vi "pulse amplitude fitter.vi"() -> ()   [LabVIEW 2016]
uses:
  <vilib>/Analysis/4window.llb/Hanning Window (DBL).vi
  <vilib>/Analysis/baseanly.llb/Real Dot Product.vi
  <vilib>/Analysis/baseanly.llb/Mean (DBL).vi
  <vilib>/Analysis/4window.llb/AllCosWindow (DBL).vi
  subs/path list.vi
  subs/global mass.vi
  <vilib>/Analysis/NI_AALPro.lvlib
  <vilib>/Analysis/NI_AALBase.lvlib
panel:
  in  "experiment":u16(ring) items=["2D SdH", "2D dHvA (dM/dt)", "2D dHvA (dM/dB)", "2D dHvA (M)", "2D dHvA (torque)", "3D SdH", "3D dHvA (dM/dt)", "3D dHvA (dM/dB)", "3D dHvA (M)", "3D dHvA (torque)"]
  in  "save parameters?":bool
  in  "save plots?":bool
  in  "format":string="%.6e"
  in  "?":bool
  in  "renomalise\namplitudes?":dbl[](array[numeric]) format="%.2f"
  out "fitted intercept":dbl[][](array[numeric]) format="%.2f"
  out "fitted m* over all (1/b)":dbl[](array[numeric]) format="%.2f"
  out "fitted gamma":dbl[][](array[numeric]) format="%.2f"
  in  "mass constant":dbl=1.0 format="%.2f"
  in  "Dingle plot mass option":u16(ring) items=["single fitted value", "field dependent", "use mass constant"]
  out "fitted m*":dbl[][](array[numeric]) format="%.2f"
  out "plot parameters":string="1/B   F   m*"
  in  "selection":u16(ring) items=["amp. vs. temperature T", "amp. vs. 1/B"]
  in  "no. points in 1/B":u16(ring) items=["1", "3", "7", "15", "31", "63", "127"]
  in  "frequencies":dbl[](array[numeric]) format="%.2f"
  in  "temperatures":dbl[](array[numeric]) format="%.2f"
  out "plotted data":cluster{"temperatures":dbl[], dbl[]}[](graph)
  in  "type of interpolation":u16(ring) items=["linear", "cubic spline", "polynomial"]
  in  "no. 1/B interpolation points":u16(ring) items=["1024", "2048", "4096", "8192", "16384", "32768"]
  in  "y domain":u16(ring) items=["channel A"]
  in  "x domain":u16(ring) items=["1/B (rising field)", "1/B (falling field)", "1/B (rising field + falling field)", "1/B (rising field - falling field)"]
  # "#\n0\n1\n2\n3\n4\n5\n6\n7\n8\n9\n10\n11\n12\n13\n14\n15\n16\n17\n18\n19\n20\n21\n22\n23\n24\n25\n26\n27\n28\n29\n30"
  # "1/B"
  # "T"
  # "F"
  # "F"
  # "T"
  # "F"
  # "F"
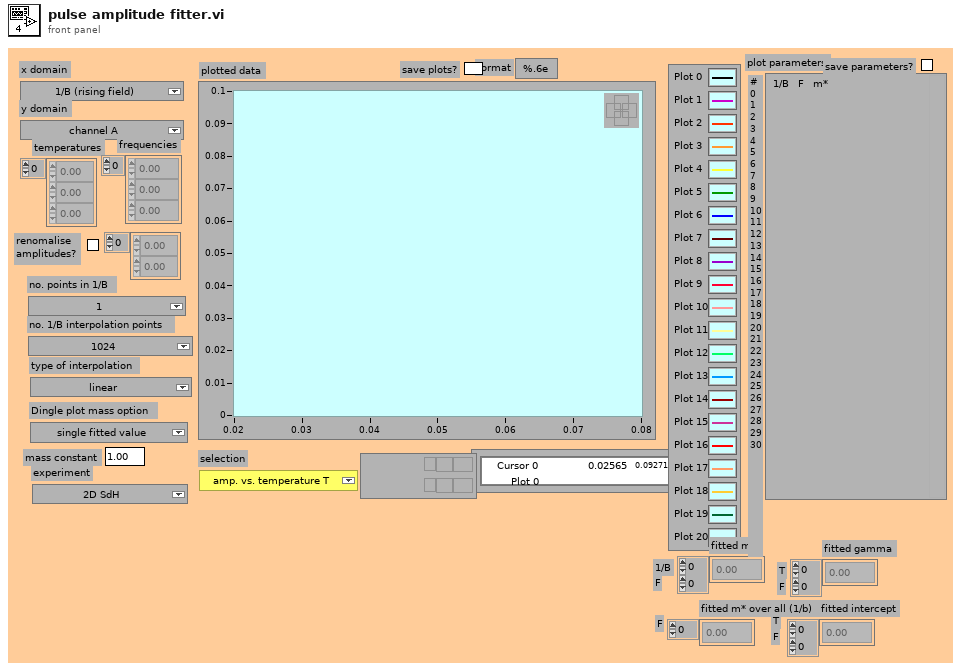
[diagram p1: front panel]
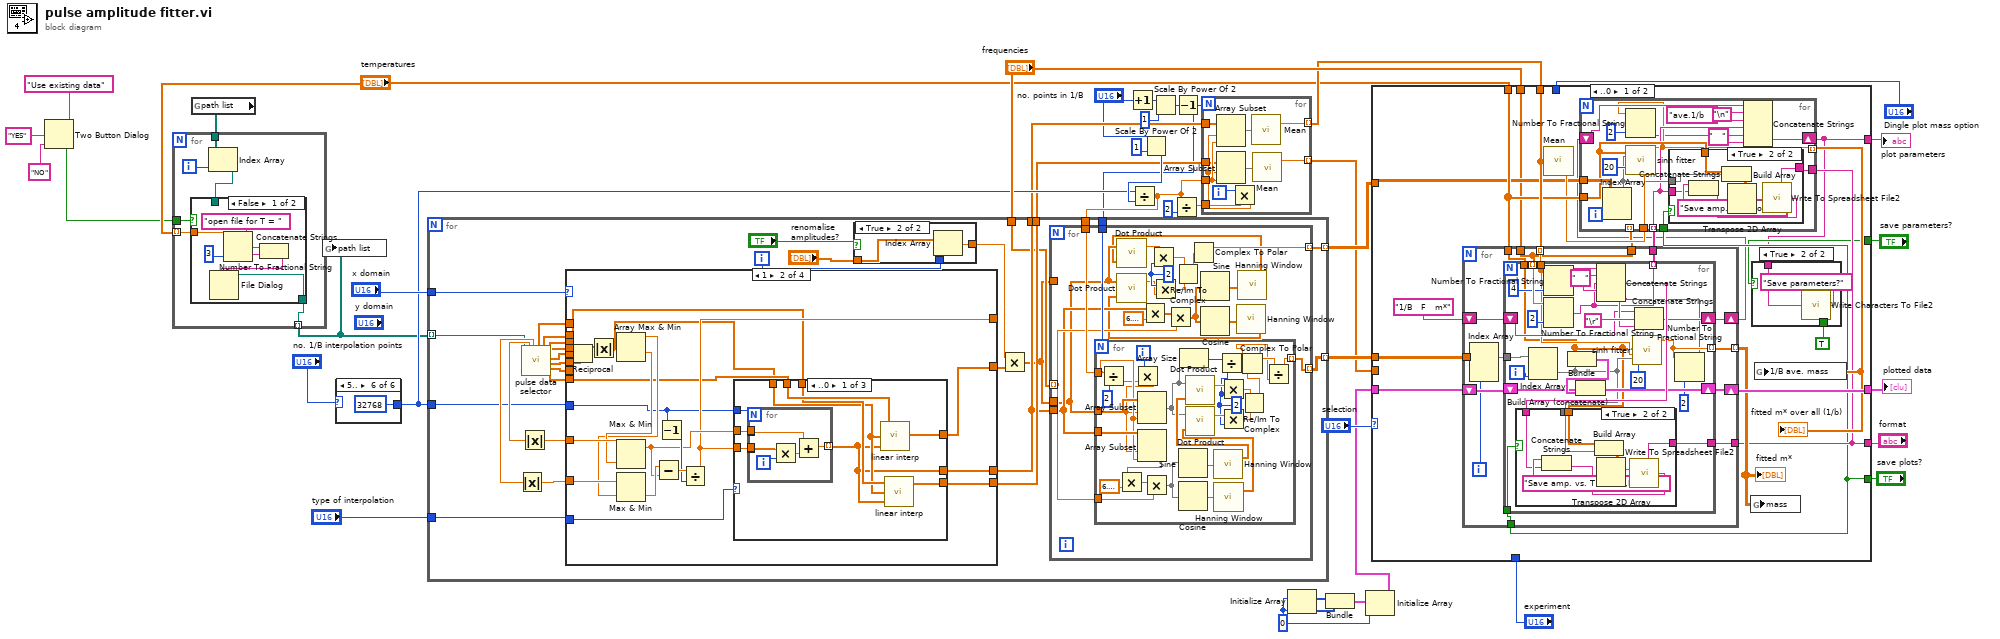
[diagram p0: block diagram]
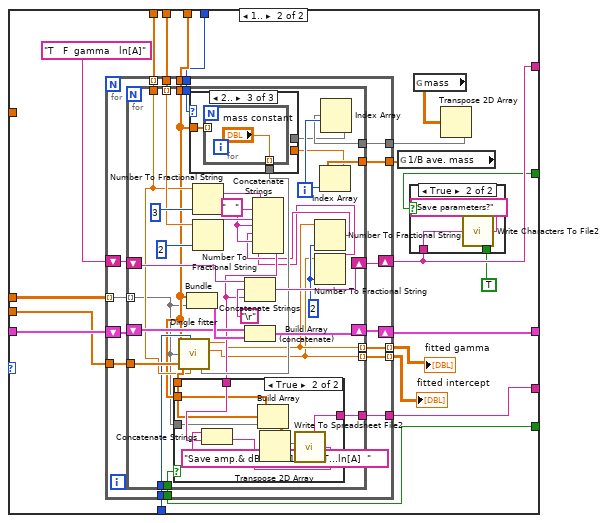
[diagram p6: hidden frame]
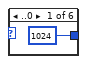
[diagram p11: hidden frame]
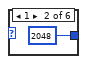
[diagram p12: hidden frame]
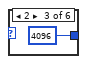
[diagram p13: hidden frame]
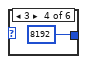
[diagram p14: hidden frame]
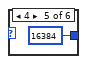
[diagram p15: hidden frame]
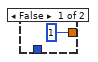
[diagram p16: hidden frame]
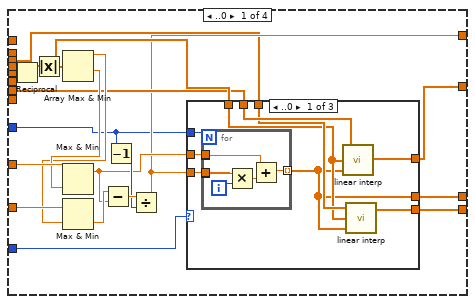
[diagram p17: hidden frame]
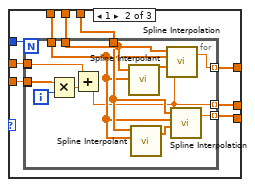
[diagram p18: hidden frame]
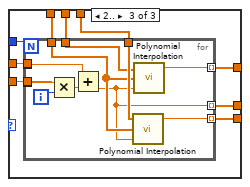
[diagram p19: hidden frame]
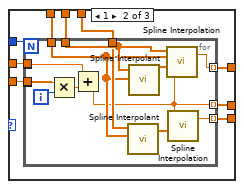
[diagram p20: hidden frame]
diagram:
  w23 = 0
  n1 = Two Button Dialog(message="Use existing data", 1:"NO", 2:"YES") -> (T button?=w8:bool)
  n2 = global read "path list.vi" "path list"() -> (w12:path[])
  n3 = for {
    tunnel: "temperatures" -> [w46] mode=indexing
    tunnel: [w45] -> w13 mode=indexing
    tunnel: w12 -> [w43]
    tunnel: w8 -> [w44]
    i -> [w42]
    n4 = Index Array(array=w43, index=w42) -> (element=w41:path)
    n5 = case shown="False" w44 {
      tunnel: w46 -> [w48 _]
      tunnel: [w47 w53] -> w45
      tunnel: w41 -> [_ w53]
      frame False {
        n6 = Number To Fractional String(number=w48, precision (6)=3) -> (F-format string=w51:string)  [unwired: 2 in]
        n7 = Concatenate Strings("open file for T = ", w51) -> (w52:string)
        n8 = File Dialog(7:w52) -> (3:w47:path)  [unwired: 6 in, 3 out]
      }
      frame True {
      }
    }
  }
  n9 = global write "path list.vi" "path list"(w13) -> ()
  n10 = case shown="5.." "no. 1/B interpolation points" {
    tunnel: [1024 2048 4096 8192 16384 32768] -> w32
    frame ..0 {
    }
    frame 1 {
    }
    frame 2 {
    }
    frame 3 {
    }
    frame 4 {
    }
    frame 5.. {
    }
  }
  n11 = Increment(x="no. points in 1/B") -> (x+1=w36:u16)
  n12 = Scale By Power Of 2(n="no. points in 1/B", x=1) -> (x*2^n=w34:i32)
  n13 = Divide(x=w32, y=w34) -> (x/y=w31:dbl)
  n14 = Scale By Power Of 2(n=w36, x=1) -> (x*2^n=w35:i32)
  n15 = Divide(x=w31, y=2) -> (x/y=w29:dbl)
  n16 = Decrement(x=w35) -> (x-1=w16:i32)
  n17 = for {
    tunnel: "x domain" -> [w70]
    tunnel: w32 -> [w78]
    tunnel: "type of interpolation" -> [w77]
    tunnel: [w76] -> w25 mode=indexing
    tunnel: "frequencies" -> [w67]
    tunnel: w31 -> [w73]
    tunnel: [w68] -> w28
    tunnel: [w72] -> w27
    tunnel: w16 -> [w71]
    tunnel: w13 -> [w69] mode=indexing
    tunnel: [w66] -> w7 mode=indexing
    i -> [w63]
    n18 = call "pulse data selector.vi"("file path (dialog if empty)"=w69) -> ("1/B start interpolation"=w83:dbl, "1/B end interpolation"=w84:dbl, "time rising"=w79:dbl[], "time falling"=w80:dbl[], "dB/dt rising"=w75:dbl[], "dB/dt falling"=w74:dbl[], "B rising"=w87:dbl[], "B falling"=w88:dbl[], "ch A rising"=w81:dbl[], "ch A falling"=w82:dbl[])  [unwired: 6 in, 3 out]
    n19 = Absolute Value(x=w84) -> (abs(x)=w86:dbl)
    n20 = Absolute Value(x=w83) -> (abs(x)=w85:dbl)
    n21 = case shown="1" w70 {
      tunnel: w79 -> [_ _ _ _]
      tunnel: w80 -> [_ _ _ _]
      tunnel: w81 -> [w147 _ w298 w430]
      tunnel: w82 -> [_ w219 w299 w431]
      tunnel: [w146 w222 w290 w422] -> w62
      tunnel: [w145 w221 w294 w426] -> _
      tunnel: w78 -> [w140 w213 w286 w418]
      tunnel: w85 -> [w157 w231 w301 w433]
      tunnel: w86 -> [w155 w229 w300 w432]
      tunnel: w87 -> [w150 _ w296 w428]
      tunnel: w88 -> [_ w220 w303 w435]
      tunnel: w77 -> [w149 w224 w302 w434]
      tunnel: [w143 w216 w289 w421] -> w68
      tunnel: w75 -> [w142 _ _ _]
      tunnel: [w141 w215 w287 w419] -> w72
      tunnel: w74 -> [_ w214 _ _]
      frame ..0 {
        n22 = Reciprocal(x=w150) -> (1/x=w144:dbl[])
        n23 = Absolute Value(x=w144) -> (abs(x)=w158:dbl[])
        n24 = Array Max & Min(array=w158) -> (max value=w154:dbl, min value=w156:dbl)  [unwired: 2 out]
        n25 = Max & Min(x=w157, y=w156) -> (max(x,y)=w148:dbl)  [unwired: 1 out]
        n26 = Max & Min(x=w155, y=w154) -> (min(x,y)=w153:dbl)  [unwired: 1 out]
        n27 = Subtract(x=w153, y=w148) -> (x-y=w152:dbl)
        n28 = Decrement(x=w140) -> (x-1=w151:i32)
        n29 = Divide(x=w152, y=w151) -> (x/y=w145:dbl)
        n30 = case shown="..0" w149 {
          tunnel: w140 -> [w167 w181 w202]
          tunnel: w148 -> [w166 w180 w201]
          tunnel: w145 -> [w165 w179 w200]
          tunnel: w158 -> [w161 w178 w199]
          tunnel: w147 -> [w164 w177 w198]
          tunnel: [w163 w176 w197] -> w146
          tunnel: [w160 w175 w196] -> w143
          tunnel: w142 -> [w162 w174 w195]
          tunnel: [w159 w173 w194] -> w141
          frame ..0 {
            n31 = for {
              N: w167 -> [_]
              tunnel: [w169] -> _ mode=indexing
              tunnel: [w170] -> _ mode=indexing
              tunnel: w166 -> [w170]
              tunnel: w165 -> [w169]
              tunnel: [w168] -> w160 mode=indexing
              i -> [w172]
              n32 = Multiply(x=w169, y=w172) -> (x*y=w171:dbl)
              n33 = Add(x=w170, y=w171) -> (x+y=w168:dbl)
            }
            n34 = call "linear interp.vi"("x array"=w160, "X data"=w161, "Y data"=w164) -> ("y"=w163:dbl[])
            n35 = call "linear interp.vi"("x array"=w160, "X data"=w161, "Y data"=w162) -> ("y"=w159:dbl[])
          }
          frame 1 {
            n36 = for {
              N: w181 -> [_]
              tunnel: [w190] -> _ mode=indexing
              tunnel: [w191] -> _ mode=indexing
              tunnel: w180 -> [w191]
              tunnel: w179 -> [w190]
              tunnel: w178 -> [w185]
              tunnel: w177 -> [w189]
              tunnel: [w187] -> w176 mode=indexing
              tunnel: [w182] -> w175 mode=indexing
              tunnel: w174 -> [w186]
              tunnel: [w183] -> w173 mode=indexing
              i -> [w193]
              n37 = Multiply(x=w190, y=w193) -> (x*y=w192:dbl)
              n38 = Add(x=w191, y=w192) -> (x+y=w182:dbl)
              n39 = call <vilib>:"Spline Interpolant.vi"("X"=w185, "Y"=w189) -> ("Interpolant"=w188:dbl[])  [unwired: 2 in, 1 out]
              n40 = call <vilib>:"Spline Interpolant.vi"("X"=w185, "Y"=w186) -> ("Interpolant"=w184:dbl[])  [unwired: 2 in, 1 out]
              n41 = call <vilib>:"Spline Interpolation.vi"("x value"=w182, "Interpolant"=w188, "X"=w185, "Y"=w189) -> ("interpolation value"=w187:dbl)  [unwired: 1 out]
              n42 = call <vilib>:"Spline Interpolation.vi"("x value"=w182, "Interpolant"=w184, "X"=w185, "Y"=w186) -> ("interpolation value"=w183:dbl)  [unwired: 1 out]
            }
          }
          frame 2.. {
            n43 = for {
              N: w202 -> [_]
              tunnel: [w209] -> _ mode=indexing
              tunnel: [w210] -> _ mode=indexing
              tunnel: w201 -> [w210]
              tunnel: w200 -> [w209]
              tunnel: w199 -> [w205]
              tunnel: w198 -> [w206]
              tunnel: [w208] -> w197 mode=indexing
              tunnel: [w204] -> w196 mode=indexing
              tunnel: w195 -> [w207]
              tunnel: [w203] -> w194 mode=indexing
              i -> [w212]
              n44 = Multiply(x=w209, y=w212) -> (x*y=w211:dbl)
              n45 = Add(x=w210, y=w211) -> (x+y=w204:dbl)
              n46 = call <vilib>:"Polynomial Interpolation.vi"("x value"=w204, "X"=w205, "Y"=w207) -> ("interpolation value"=w203:dbl)  [unwired: 2 out]
              n47 = call <vilib>:"Polynomial Interpolation.vi"("x value"=w204, "X"=w205, "Y"=w206) -> ("interpolation value"=w208:dbl)  [unwired: 2 out]
            }
          }
        }
      }
      frame 1 {
        n48 = Reciprocal(x=w220) -> (1/x=w218:dbl[])
        n49 = Absolute Value(x=w218) -> (abs(x)=w217:dbl[])
        n50 = Array Max & Min(array=w217) -> (max value=w228:dbl, min value=w230:dbl)  [unwired: 2 out]
        n51 = Max & Min(x=w231, y=w230) -> (max(x,y)=w223:dbl)  [unwired: 1 out]
        n52 = Max & Min(x=w229, y=w228) -> (min(x,y)=w227:dbl)  [unwired: 1 out]
        n53 = Subtract(x=w227, y=w223) -> (x-y=w226:dbl)
        n54 = Decrement(x=w213) -> (x-1=w225:i32)
        n55 = Divide(x=w226, y=w225) -> (x/y=w221:dbl)
        n56 = case shown="..0" w224 {
          tunnel: w213 -> [w240 w254 w275]
          tunnel: w223 -> [w239 w253 w274]
          tunnel: w221 -> [w238 w252 w273]
          tunnel: w217 -> [w233 w251 w272]
          tunnel: w219 -> [w237 w250 w271]
          tunnel: [w236 w249 w270] -> w222
          tunnel: [w232 w248 w269] -> w216
          tunnel: [w235 w247 w268] -> w215
          tunnel: w214 -> [w234 w246 w267]
          frame ..0 {
            n57 = for {
              N: w240 -> [_]
              tunnel: [w242] -> _ mode=indexing
              tunnel: [w243] -> _ mode=indexing
              tunnel: w239 -> [w243]
              tunnel: w238 -> [w242]
              tunnel: [w241] -> w232 mode=indexing
              i -> [w245]
              n58 = Multiply(x=w242, y=w245) -> (x*y=w244:dbl)
              n59 = Add(x=w243, y=w244) -> (x+y=w241:dbl)
            }
            n60 = call "linear interp.vi"("x array"=w232, "X data"=w233, "Y data"=w237) -> ("y"=w236:dbl[])
            n61 = call "linear interp.vi"("x array"=w232, "X data"=w233, "Y data"=w234) -> ("y"=w235:dbl[])
          }
          frame 1 {
            n62 = for {
              N: w254 -> [_]
              tunnel: [w263] -> _ mode=indexing
              tunnel: [w264] -> _ mode=indexing
              tunnel: w253 -> [w264]
              tunnel: w252 -> [w263]
              tunnel: w251 -> [w256]
              tunnel: w250 -> [w262]
              tunnel: [w260] -> w249 mode=indexing
              tunnel: [w255] -> w248 mode=indexing
              tunnel: [w259] -> w247 mode=indexing
              tunnel: w246 -> [w257]
              i -> [w266]
              n63 = Multiply(x=w263, y=w266) -> (x*y=w265:dbl)
              n64 = Add(x=w264, y=w265) -> (x+y=w255:dbl)
              n65 = call <vilib>:"Spline Interpolant.vi"("X"=w256, "Y"=w257) -> ("Interpolant"=w258:dbl[])  [unwired: 2 in, 1 out]
              n66 = call <vilib>:"Spline Interpolant.vi"("X"=w256, "Y"=w262) -> ("Interpolant"=w261:dbl[])  [unwired: 2 in, 1 out]
              n67 = call <vilib>:"Spline Interpolation.vi"("x value"=w255, "Interpolant"=w261, "X"=w256, "Y"=w262) -> ("interpolation value"=w260:dbl)  [unwired: 1 out]
              n68 = call <vilib>:"Spline Interpolation.vi"("x value"=w255, "Interpolant"=w258) -> ("interpolation value"=w259:dbl)  [unwired: 2 in, 1 out]
            }
          }
          frame 2.. {
            n69 = for {
              N: w275 -> [_]
              tunnel: [w282] -> _ mode=indexing
              tunnel: [w283] -> _ mode=indexing
              tunnel: w274 -> [w283]
              tunnel: w273 -> [w282]
              tunnel: w272 -> [w277]
              tunnel: w271 -> [w281]
              tunnel: [w280] -> w270 mode=indexing
              tunnel: [w276] -> w269 mode=indexing
              tunnel: [w279] -> w268 mode=indexing
              tunnel: w267 -> [w278]
              i -> [w285]
              n70 = Multiply(x=w282, y=w285) -> (x*y=w284:dbl)
              n71 = Add(x=w283, y=w284) -> (x+y=w276:dbl)
              n72 = call <vilib>:"Polynomial Interpolation.vi"("x value"=w276, "X"=w277, "Y"=w281) -> ("interpolation value"=w280:dbl)  [unwired: 2 out]
              n73 = call <vilib>:"Polynomial Interpolation.vi"("x value"=w276, "X"=w277, "Y"=w278) -> ("interpolation value"=w279:dbl)  [unwired: 2 out]
            }
          }
        }
      }
      frame 2 {
        w288 = 0
        n74 = Reciprocal(x=w303) -> (1/x=w304:dbl[])
        n75 = Reciprocal(x=w296) -> (1/x=w297:dbl[])
        n76 = Absolute Value(x=w304) -> (abs(x)=w293:dbl[])
        n77 = Absolute Value(x=w297) -> (abs(x)=w295:dbl[])
        n78 = stacked-sequence {
          tunnel: w302 -> [w307 w362]
          tunnel: w301 -> [w312 w368]
          tunnel: w300 -> [w311 w367]
          tunnel: w299 -> [_ w363]
          tunnel: w298 -> [w310 _]
          tunnel: w295 -> [w309 _]
          tunnel: w286 -> [w305 w360]
          tunnel: [_ w366] -> w292
          tunnel: [w306 _] -> w294
          tunnel: w293 -> [_ w364]
          tunnel: [w308 _] -> w291
          tunnel: [_ w361] -> w289
          frame #0 {
            n79 = Array Max & Min(array=w309) -> (max value=w314:dbl, min value=w313:dbl)  [unwired: 2 out]
            n80 = Max & Min(x=w312, y=w313) -> (max(x,y)=w315:dbl)  [unwired: 1 out]
            n81 = Max & Min(x=w311, y=w314) -> (min(x,y)=w316:dbl)  [unwired: 1 out]
            n82 = Subtract(x=w316, y=w315) -> (x-y=w318:dbl)
            n83 = Decrement(x=w305) -> (x-1=w317:i32)
            n84 = Divide(x=w318, y=w317) -> (x/y=w306:dbl)
            n85 = case shown="1" w307 {
              tunnel: w305 -> [w325 w336 w351]
              tunnel: w315 -> [w324 w335 w350]
              tunnel: w306 -> [w323 w334 w349]
              tunnel: w309 -> [w321 w333 w348]
              tunnel: w310 -> [w322 w332 w347]
              tunnel: [w319 w331 w346] -> w308
              frame ..0 {
                n86 = for {
                  N: w325 -> [_]
                  tunnel: [w327] -> _ mode=indexing
                  tunnel: [w328] -> _ mode=indexing
                  tunnel: w324 -> [w328]
                  tunnel: w323 -> [w327]
                  tunnel: [w326] -> w320 mode=indexing
                  i -> [w330]
                  n87 = Multiply(x=w327, y=w330) -> (x*y=w329:dbl)
                  n88 = Add(x=w328, y=w329) -> (x+y=w326:dbl)
                }
                n89 = call "linear interp.vi"("x array"=w320, "X data"=w321, "Y data"=w322) -> ("y"=w319:dbl[])
              }
              frame 1 {
                n90 = for {
                  N: w336 -> [_]
                  tunnel: [w342] -> _ mode=indexing
                  tunnel: [w343] -> _ mode=indexing
                  tunnel: w335 -> [w343]
                  tunnel: w334 -> [w342]
                  tunnel: w333 -> [w340]
                  tunnel: w332 -> [w341]
                  tunnel: [w337] -> w331 mode=indexing
                  i -> [w345]
                  n91 = Multiply(x=w342, y=w345) -> (x*y=w344:dbl)
                  n92 = Add(x=w343, y=w344) -> (x+y=w338:dbl)
                  n93 = call <vilib>:"Spline Interpolant.vi"("X"=w340, "Y"=w341) -> ("Interpolant"=w339:dbl[])  [unwired: 2 in, 1 out]
                  n94 = call <vilib>:"Spline Interpolation.vi"("x value"=w338, "Interpolant"=w339, "X"=w340, "Y"=w341) -> ("interpolation value"=w337:dbl)  [unwired: 1 out]
                }
              }
              frame 2.. {
                n95 = for {
                  N: w351 -> [_]
                  tunnel: [w356] -> _ mode=indexing
                  tunnel: [w357] -> _ mode=indexing
                  tunnel: w350 -> [w357]
                  tunnel: w349 -> [w356]
                  tunnel: w348 -> [w355]
                  tunnel: w347 -> [w354]
                  tunnel: [w352] -> w346 mode=indexing
                  i -> [w359]
                  n96 = Multiply(x=w356, y=w359) -> (x*y=w358:dbl)
                  n97 = Add(x=w357, y=w358) -> (x+y=w353:dbl)
                  n98 = call <vilib>:"Polynomial Interpolation.vi"("x value"=w353, "X"=w355, "Y"=w354) -> ("interpolation value"=w352:dbl)  [unwired: 2 out]
                }
              }
            }
          }
          frame #1 {
            n99 = Array Max & Min(array=w364) -> (max value=w370:dbl, min value=w369:dbl)  [unwired: 2 out]
            n100 = Max & Min(x=w368, y=w369) -> (max(x,y)=w371:dbl)  [unwired: 1 out]
            n101 = Max & Min(x=w367, y=w370) -> (min(x,y)=w372:dbl)  [unwired: 1 out]
            n102 = Subtract(x=w372, y=w371) -> (x-y=w374:dbl)
            n103 = Decrement(x=w360) -> (x-1=w373:i32)
            n104 = Divide(x=w374, y=w373) -> (x/y=w365:dbl)
            n105 = case shown="2.." w362 {
              tunnel: w360 -> [w381 w393 w409]
              tunnel: w371 -> [w380 w392 w408]
              tunnel: w365 -> [w379 w391 w407]
              tunnel: w364 -> [w377 w390 w406]
              tunnel: w363 -> [w378 w388 w405]
              tunnel: [w376 w389 w404] -> w366
              tunnel: [w375 w387 w403] -> w361
              frame ..0 {
                n106 = for {
                  N: w381 -> [_]
                  tunnel: [w383] -> _ mode=indexing
                  tunnel: [w384] -> _ mode=indexing
                  tunnel: w380 -> [w384]
                  tunnel: w379 -> [w383]
                  tunnel: [w382] -> w375 mode=indexing
                  i -> [w386]
                  n107 = Multiply(x=w383, y=w386) -> (x*y=w385:dbl)
                  n108 = Add(x=w384, y=w385) -> (x+y=w382:dbl)
                }
                n109 = call "linear interp.vi"("x array"=w375, "X data"=w377, "Y data"=w378) -> ("y"=w376:dbl[])
              }
              frame 1 {
                n110 = for {
                  N: w393 -> [_]
                  tunnel: [w399] -> _ mode=indexing
                  tunnel: [w400] -> _ mode=indexing
                  tunnel: w392 -> [w400]
                  tunnel: w391 -> [w399]
                  tunnel: w390 -> [w397]
                  tunnel: w388 -> [w398]
                  tunnel: [w395] -> w389 mode=indexing
                  tunnel: [w394] -> w387 mode=indexing
                  i -> [w402]
                  n111 = Multiply(x=w399, y=w402) -> (x*y=w401:dbl)
                  n112 = Add(x=w400, y=w401) -> (x+y=w394:dbl)
                  n113 = call <vilib>:"Spline Interpolant.vi"("X"=w397, "Y"=w398) -> ("Interpolant"=w396:dbl[])  [unwired: 2 in, 1 out]
                  n114 = call <vilib>:"Spline Interpolation.vi"("x value"=w394, "Interpolant"=w396, "X"=w397, "Y"=w398) -> ("interpolation value"=w395:dbl)  [unwired: 1 out]
                }
              }
              frame 2.. {
                n115 = for {
                  N: w409 -> [_]
                  tunnel: [w414] -> _ mode=indexing
                  tunnel: [w415] -> _ mode=indexing
                  tunnel: w408 -> [w415]
                  tunnel: w407 -> [w414]
                  tunnel: w406 -> [w413]
                  tunnel: w405 -> [w412]
                  tunnel: [w411] -> w404 mode=indexing
                  tunnel: [w410] -> w403 mode=indexing
                  i -> [w417]
                  n116 = Multiply(x=w414, y=w417) -> (x*y=w416:dbl)
                  n117 = Add(x=w415, y=w416) -> (x+y=w410:dbl)
                  n118 = call <vilib>:"Polynomial Interpolation.vi"("x value"=w410, "X"=w413, "Y"=w412) -> ("interpolation value"=w411:dbl)  [unwired: 2 out]
                }
              }
            }
          }
        }
        n119 = Add(x=w291, y=w292) -> (x+y=w290:dbl[])
        n120 = Initialize Array(w288, w288) -> (w287:i32[])
      }
      frame 3.. {
        w420 = 0
        n121 = Reciprocal(x=w435) -> (1/x=w436:dbl[])
        n122 = Reciprocal(x=w428) -> (1/x=w429:dbl[])
        n123 = Absolute Value(x=w436) -> (abs(x)=w425:dbl[])
        n124 = Absolute Value(x=w429) -> (abs(x)=w427:dbl[])
        n125 = stacked-sequence {
          tunnel: w434 -> [w437 w494]
          tunnel: w433 -> [w444 w500]
          tunnel: w432 -> [w443 w499]
          tunnel: w431 -> [_ w495]
          tunnel: w430 -> [w442 _]
          tunnel: w427 -> [w441 _]
          tunnel: w418 -> [w440 w492]
          tunnel: [_ w498] -> w424
          tunnel: [w438 _] -> w426
          tunnel: w425 -> [_ w496]
          tunnel: [w439 _] -> w423
          tunnel: [_ w493] -> w421
          frame #0 {
            n126 = Array Max & Min(array=w441) -> (max value=w446:dbl, min value=w445:dbl)  [unwired: 2 out]
            n127 = Max & Min(x=w444, y=w445) -> (max(x,y)=w447:dbl)  [unwired: 1 out]
            n128 = Max & Min(x=w443, y=w446) -> (min(x,y)=w448:dbl)  [unwired: 1 out]
            n129 = Subtract(x=w448, y=w447) -> (x-y=w450:dbl)
            n130 = Decrement(x=w440) -> (x-1=w449:i32)
            n131 = Divide(x=w450, y=w449) -> (x/y=w438:dbl)
            n132 = case shown="1" w437 {
              tunnel: w440 -> [w457 w468 w483]
              tunnel: w447 -> [w456 w467 w482]
              tunnel: w438 -> [w455 w466 w481]
              tunnel: w441 -> [w453 w465 w480]
              tunnel: w442 -> [w454 w464 w479]
              tunnel: [w451 w463 w478] -> w439
              frame ..0 {
                n133 = for {
                  N: w457 -> [_]
                  tunnel: [w459] -> _ mode=indexing
                  tunnel: [w460] -> _ mode=indexing
                  tunnel: w456 -> [w460]
                  tunnel: w455 -> [w459]
                  tunnel: [w458] -> w452 mode=indexing
                  i -> [w462]
                  n134 = Multiply(x=w459, y=w462) -> (x*y=w461:dbl)
                  n135 = Add(x=w460, y=w461) -> (x+y=w458:dbl)
                }
                n136 = call "linear interp.vi"("x array"=w452, "X data"=w453, "Y data"=w454) -> ("y"=w451:dbl[])
              }
              frame 1 {
                n137 = for {
                  N: w468 -> [_]
                  tunnel: [w474] -> _ mode=indexing
                  tunnel: [w475] -> _ mode=indexing
                  tunnel: w467 -> [w475]
                  tunnel: w466 -> [w474]
                  tunnel: w465 -> [w472]
                  tunnel: w464 -> [w473]
                  tunnel: [w469] -> w463 mode=indexing
                  i -> [w477]
                  n138 = Multiply(x=w474, y=w477) -> (x*y=w476:dbl)
                  n139 = Add(x=w475, y=w476) -> (x+y=w470:dbl)
                  n140 = call <vilib>:"Spline Interpolant.vi"("X"=w472, "Y"=w473) -> ("Interpolant"=w471:dbl[])  [unwired: 2 in, 1 out]
                  n141 = call <vilib>:"Spline Interpolation.vi"("x value"=w470, "Interpolant"=w471, "X"=w472, "Y"=w473) -> ("interpolation value"=w469:dbl)  [unwired: 1 out]
                }
              }
              frame 2.. {
                n142 = for {
                  N: w483 -> [_]
                  tunnel: [w488] -> _ mode=indexing
                  tunnel: [w489] -> _ mode=indexing
                  tunnel: w482 -> [w489]
                  tunnel: w481 -> [w488]
                  tunnel: w480 -> [w487]
                  tunnel: w479 -> [w486]
                  tunnel: [w484] -> w478 mode=indexing
                  i -> [w491]
                  n143 = Multiply(x=w488, y=w491) -> (x*y=w490:dbl)
                  n144 = Add(x=w489, y=w490) -> (x+y=w485:dbl)
                  n145 = call <vilib>:"Polynomial Interpolation.vi"("x value"=w485, "X"=w487, "Y"=w486) -> ("interpolation value"=w484:dbl)  [unwired: 2 out]
                }
              }
            }
          }
          frame #1 {
            n146 = Array Max & Min(array=w496) -> (max value=w502:dbl, min value=w501:dbl)  [unwired: 2 out]
            n147 = Max & Min(x=w500, y=w501) -> (max(x,y)=w503:dbl)  [unwired: 1 out]
            n148 = Max & Min(x=w499, y=w502) -> (min(x,y)=w504:dbl)  [unwired: 1 out]
            n149 = Subtract(x=w504, y=w503) -> (x-y=w506:dbl)
            n150 = Decrement(x=w492) -> (x-1=w505:i32)
            n151 = Divide(x=w506, y=w505) -> (x/y=w497:dbl)
            n152 = case shown="..0" w494 {
              tunnel: w492 -> [w513 w525 w541]
              tunnel: w503 -> [w512 w524 w540]
              tunnel: w497 -> [w511 w523 w539]
              tunnel: w496 -> [w509 w522 w538]
              tunnel: w495 -> [w510 w521 w537]
              tunnel: [w508 w520 w536] -> w498
              tunnel: [w507 w519 w535] -> w493
              frame ..0 {
                n153 = for {
                  N: w513 -> [_]
                  tunnel: [w515] -> _ mode=indexing
                  tunnel: [w516] -> _ mode=indexing
                  tunnel: w512 -> [w516]
                  tunnel: w511 -> [w515]
                  tunnel: [w514] -> w507 mode=indexing
                  i -> [w518]
                  n154 = Multiply(x=w515, y=w518) -> (x*y=w517:dbl)
                  n155 = Add(x=w516, y=w517) -> (x+y=w514:dbl)
                }
                n156 = call "linear interp.vi"("x array"=w507, "X data"=w509, "Y data"=w510) -> ("y"=w508:dbl[])
              }
              frame 1 {
                n157 = for {
                  N: w525 -> [_]
                  tunnel: [w531] -> _ mode=indexing
                  tunnel: [w532] -> _ mode=indexing
                  tunnel: w524 -> [w532]
                  tunnel: w523 -> [w531]
                  tunnel: w522 -> [w529]
                  tunnel: w521 -> [w530]
                  tunnel: [w527] -> w520 mode=indexing
                  tunnel: [w526] -> w519 mode=indexing
                  i -> [w534]
                  n158 = Multiply(x=w531, y=w534) -> (x*y=w533:dbl)
                  n159 = Add(x=w532, y=w533) -> (x+y=w526:dbl)
                  n160 = call <vilib>:"Spline Interpolant.vi"("X"=w529, "Y"=w530) -> ("Interpolant"=w528:dbl[])  [unwired: 2 in, 1 out]
                  n161 = call <vilib>:"Spline Interpolation.vi"("x value"=w526, "Interpolant"=w528, "X"=w529, "Y"=w530) -> ("interpolation value"=w527:dbl)  [unwired: 1 out]
                }
              }
              frame 2.. {
                n162 = for {
                  N: w541 -> [_]
                  tunnel: [w546] -> _ mode=indexing
                  tunnel: [w547] -> _ mode=indexing
                  tunnel: w540 -> [w547]
                  tunnel: w539 -> [w546]
                  tunnel: w538 -> [w545]
                  tunnel: w537 -> [w544]
                  tunnel: [w543] -> w536 mode=indexing
                  tunnel: [w542] -> w535 mode=indexing
                  i -> [w549]
                  n163 = Multiply(x=w546, y=w549) -> (x*y=w548:dbl)
                  n164 = Add(x=w547, y=w548) -> (x+y=w542:dbl)
                  n165 = call <vilib>:"Polynomial Interpolation.vi"("x value"=w542, "X"=w545, "Y"=w544) -> ("interpolation value"=w543:dbl)  [unwired: 2 out]
                }
              }
            }
          }
        }
        n166 = Subtract(x=w423, y=w424) -> (x-y=w422:dbl[])
        n167 = Initialize Array(w420, w420) -> (w419:i32[])
      }
    }
    n168 = case shown="True" "?" {
      tunnel: "renomalise\namplitudes?" -> [_ w92]
      tunnel: [1 w91] -> w61
      tunnel: w63 -> [_ w90]
      frame False {
      }
      frame True {
        n169 = Index Array(array=w92, index=w90) -> (element=w91:dbl)
      }
    }
    n170 = Multiply(x=w61, y=w62) -> (x*y=w60:dbl[])
    n171 = for {
      tunnel: w67 -> [w106] mode=indexing
      tunnel: w60 -> [w102]
      tunnel: w68 -> [w103]
      tunnel: [w112] -> w76 mode=indexing
      tunnel: w71 -> [w110]
      tunnel: w73 -> [w111]
      tunnel: w60 -> [_]
      tunnel: [w95] -> w66 mode=indexing
      w101 = 2
      n172 = for {
        N: w110 -> [_]
        tunnel: w111 -> [w136]
        tunnel: w102 -> [w138]
        tunnel: w103 -> [w137]
        tunnel: w106 -> [w129]
        tunnel: [w117] -> w112 mode=indexing
        i -> [w135]
        w113 = 2
        n173 = Divide(x=w136, y=2) -> (x/y=w134:dbl)
        n174 = Multiply(x=w135, y=w134) -> (x*y=w133:dbl)
        n175 = Array Subset(array=w138, index=w133, length=w136) -> (w116:dbl[])
        n176 = Array Subset(array=w137, index=w133, length=w136) -> (w132:dbl[])
        n177 = Multiply(x=w132, y=6.283185307179586) -> (x*y=w130:dbl[])
        n178 = Multiply(x=w130, y=w129) -> (x*y=w128:dbl[])
        n179 = Sine(x=w128) -> (sin(x)=w127:dbl[])
        n180 = Cosine(x=w128) -> (cos(x)=w126:dbl[])
        n181 = Array Size(array=w116) -> (size(s)=w114:i32)
        n182 = call-poly <vilib>:"Hanning Window.vi"("X"=w127) -> ("Windowed X"=w125:dbl[])  [unwired: 1 out]
        n183 = call-poly <vilib>:"Dot Product.vi"("Y Vector"=w125, "X Vector"=w116) -> ("X * Y"=w123:dbl)  [unwired: 1 out]
        n184 = call-poly <vilib>:"Hanning Window.vi"("X"=w126) -> ("Windowed X"=w124:dbl[])  [unwired: 1 out]
        n185 = call-poly <vilib>:"Dot Product.vi"("Y Vector"=w124, "X Vector"=w116) -> ("X * Y"=w122:dbl)  [unwired: 1 out]
        n186 = Divide(x=w114, y=w113) -> (x/y=w115:dbl)
        n187 = Multiply(x=w123, y=w113) -> (x*y=w121:dbl)
        n188 = Multiply(x=w122, y=w113) -> (x*y=w120:dbl)
        n189 = Re/Im To Complex(1:w120, 2:w121) -> (0:w119:cdb)
        n190 = Complex To Polar(r * e^(i*theta)=w119) -> (r=w118:dbl)  [unwired: 1 out]
        n191 = Divide(x=w118, y=w115) -> (x/y=w117:dbl)
      }
      n192 = Multiply(x=w103, y=6.283185307179586) -> (x*y=w108:dbl[])
      n193 = Multiply(x=w108, y=w106) -> (x*y=w107:dbl[])
      n194 = Sine(x=w107) -> (sin(x)=w105:dbl[])
      n195 = Cosine(x=w107) -> (cos(x)=w104:dbl[])
      n196 = call-poly <vilib>:"Hanning Window.vi"("X"=w104) -> ("Windowed X"=w93:dbl[])  [unwired: 1 out]
      n197 = call-poly <vilib>:"Dot Product.vi"("Y Vector"=w93, "X Vector"=w102) -> ("X * Y"=w99:dbl)  [unwired: 1 out]
      n198 = Multiply(x=w101, y=w99) -> (x*y=w98:dbl)
      n199 = call-poly <vilib>:"Hanning Window.vi"("X"=w105) -> ("Windowed X"=w94:dbl[])  [unwired: 1 out]
      n200 = call-poly <vilib>:"Dot Product.vi"("Y Vector"=w94, "X Vector"=w102) -> ("X * Y"=w100:dbl)  [unwired: 1 out]
      n201 = Multiply(x=w100, y=w101) -> (x*y=w97:dbl)
      n202 = Re/Im To Complex(1:w98, 2:w97) -> (0:w96:cdb)
      n203 = Complex To Polar(r * e^(i*theta)=w96) -> (r=w95:dbl)  [unwired: 1 out]
    }
  }
  n204 = for {
    N: w16 -> [_]
    tunnel: w31 -> [w559]
    tunnel: w29 -> [w557]
    tunnel: w28 -> [w555]
    tunnel: w27 -> [w554]
    tunnel: [w551] -> w24 mode=indexing
    tunnel: [w550] -> w6 mode=indexing
    i -> [w558]
    n205 = Multiply(x=w558, y=w557) -> (x*y=w556:dbl)
    n206 = Array Subset(array=w555, index=w556, length=w559) -> (w553:dbl[])
    n207 = Array Subset(array=w554, index=w556, length=w559) -> (w552:dbl[])
    n208 = call-poly <vilib>:"Mean.vi"("X"=w553) -> ("mean"=w551:dbl)  [unwired: 1 out]
    n209 = call-poly <vilib>:"Mean.vi"("X"=w552) -> ("mean"=w550:dbl)  [unwired: 1 out]
  }
  n210 = Initialize Array(w23, w23) -> (w22:i32[])
  n211 = Bundle(w22, w22) -> (w21:cluster{i32[], i32[]})  [unwired: 1 in]
  n212 = Initialize Array(w21, w23) -> (w20:cluster{i32[], i32[]}[])
  n213 = case shown="..0" "selection" {
    tunnel: w25 -> [w572 w658]
    tunnel: "temperatures" -> [w574 w672]
    tunnel: "frequencies" -> [w568 w671]
    tunnel: w24 -> [w575 w670]
    tunnel: w20 -> [w577 w668]
    tunnel: [w576 w667] -> w19
    tunnel: [w561 w655] -> w15
    tunnel: w7 -> [w571 _]
    tunnel: w6 -> [_ w666]
    tunnel: "experiment" -> [_ w665]
    tunnel: "Dingle plot mass option" -> [_ w662]
    tunnel: "format" -> [w566 w657]
    tunnel: "save plots?" -> [w565 w656]
    tunnel: "save parameters?" -> [w563 w654]
    frame ..0 {
      n214 = for {
        tunnel: w572 -> [w618]
        tunnel: w574 -> [w620]
        tunnel: w568 -> [w610]
        tunnel: w575 -> [w619] mode=indexing
        shift-right: [w615] -> w562
        shift-left: "1/B   F   m*" -> [w616]
        shift-right: [w613] -> w576
        shift-left: w577 -> [w614]
        tunnel: [w612] -> w570 mode=indexing
        tunnel: [w610] -> w567
        tunnel: w566 -> [w609]
        tunnel: w565 -> [w608]
        tunnel: [w607] -> w564
        i -> [w611]
        n215 = Index Array(array=w618, index (dim 2)=w611) -> (element=w617:dbl[][])  [unwired: 2 in]
        n216 = for {
          tunnel: w620 -> [w625]
          tunnel: w610 -> [w642] mode=indexing
          tunnel: w619 -> [w632]
          tunnel: w617 -> [w643]
          shift-right: [w633] -> w613
          shift-left: w614 -> [w638]
          shift-right: [w629] -> w615
          shift-left: w616 -> [w634]
          tunnel: [w623] -> w612 mode=indexing
          tunnel: w609 -> [w628]
          tunnel: w608 -> [w627]
          tunnel: [w624] -> w607 mode=indexing
          i -> [w630]
          w635 = "   "
          n217 = Index Array(array=w643, index (col)=w630) -> (element=w626:dbl[])  [unwired: 1 in]
          n218 = Number To Fractional String(number=w632, precision (6)=4) -> (F-format string=w639:string)  [unwired: 2 in]
          n219 = Number To Fractional String(number=w642, precision (6)=2) -> (F-format string=w624:string)  [unwired: 2 in]
          n220 = Bundle("temperatures"=w625, w626) -> (w644:cluster{"temperatures":dbl[], dbl[]})  [unwired: 1 in]
          n221 = Build Array (concatenate)(w638, w644) -> (w633:cluster{"temperatures":dbl[], dbl[]}[])
          n222 = call "sinh fitter.vi"("iterations"=20, "1/B"=w632, "amp."=w626, "T"=w625) -> ("m*"=w623:dbl)  [unwired: 2 out]
          n223 = Number To Fractional String(number=w623, precision (6)=2) -> (F-format string=w621:string)  [unwired: 2 in]
          n224 = Concatenate Strings(w639, w635, w624, w635, w621) -> (w636:string)
          n225 = case shown="True" w627 {
            tunnel: w636 -> [_ w651]
            tunnel: w628 -> [_ w648]
            tunnel: w626 -> [_ w645]
            tunnel: w625 -> [_ w646]
            frame False {
            }
            frame True {
              n226 = Concatenate Strings("Save amp. vs. T for 1/B,F,m* ", w651) -> (w647:string)
              n227 = Build Array(w646, w645) -> (w650:dbl[][])
              n228 = Transpose 2D Array(2D array=w650) -> (transposed array=w649:dbl[][])
              n229 = call "Write To Spreadsheet File2.vi"("dialogue"=w647, "format (%.3f)"=w648, "2D data"=w649) -> ()  [unwired: 5 in, 1 out]
            }
          }
          n230 = Concatenate Strings(w634, "\r", w636) -> (w629:string)
        }
      }
      "fitted m*" <- w570
      n231 = call-poly <vilib>:"Mean.vi"("X"=w575) -> ("mean"=w573:dbl)  [unwired: 1 out]
      n232 = for {
        tunnel: w571 -> [w598]
        tunnel: w574 -> [w594]
        tunnel: w573 -> [w597]
        tunnel: [w584] -> w569 mode=indexing
        tunnel: w567 -> [_] mode=indexing
        tunnel: w566 -> [w592]
        tunnel: w565 -> [w591]
        tunnel: w564 -> [w587] mode=indexing
        shift-right: [w586] -> w561
        shift-left: w562 -> [w590]
        i -> [w595]
        n233 = Index Array(array=w598, index (col)=w595) -> (element=w593:dbl[])  [unwired: 1 in]
        n234 = call "sinh fitter.vi"("iterations"=20, "1/B"=w597, "amp."=w593, "T"=w594) -> ("m*"=w584:dbl)  [unwired: 2 out]
        n235 = Number To Fractional String(number=w584, precision (6)=2) -> (F-format string=w582:string)  [unwired: 2 in]
        n236 = case shown="True" w591 {
          tunnel: w592 -> [_ w603]
          tunnel: w594 -> [_ w601]
          tunnel: w593 -> [_ w600]
          tunnel: w587 -> [_ w599]
          frame False {
          }
          frame True {
            n237 = Concatenate Strings("Save amp. vs. T for F ", w599) -> (w602:string)
            n238 = Build Array(w601, w600) -> (w605:dbl[][])
            n239 = Transpose 2D Array(2D array=w605) -> (transposed array=w604:dbl[][])
            n240 = call "Write To Spreadsheet File2.vi"("dialogue"=w602, "format (%.3f)"=w603, "2D data"=w604) -> ()  [unwired: 5 in, 1 out]
          }
        }
        n241 = Concatenate Strings(w590, "\n", "ave.1/b   ", w587, "   ", w582) -> (w586:string)
      }
      "fitted m* over all (1/b)" <- w569
      n242 = global write "global mass.vi" "mass"(w570) -> ()
      n243 = case shown="True" w563 {
        tunnel: w561 -> [_ w580]
        tunnel: TRUE -> [_ w579]
        frame False {
        }
        frame True {
          n244 = call "Write Characters To File2.vi"("convert eol? (no:F)"=w579, "prompt"="Save parameters?", "character string"=w580) -> ()  [unwired: 2 in, 1 out]
        }
      }
      n245 = global write "global mass.vi" "1/B ave. mass"(w569) -> ()
    }
    frame 1.. {
      n246 = global read "global mass.vi" "1/B ave. mass"() -> (w659:dbl[])
      n247 = global read "global mass.vi" "mass"() -> (w661:dbl[][])
      n248 = Transpose 2D Array(2D array=w661) -> (transposed array=w660:dbl[][])
      n249 = for {
        tunnel: w658 -> [w692] mode=indexing
        tunnel: w672 -> [w691] mode=indexing
        tunnel: w671 -> [w690]
        tunnel: w670 -> [w689]
        shift-right: [w687] -> w655
        shift-left: "T   F  gamma   ln[A]" -> [w688]
        shift-right: [w685] -> w667
        shift-left: w668 -> [w686]
        tunnel: w666 -> [w684]
        tunnel: w665 -> [w683]
        tunnel: [w682] -> w664 mode=indexing
        tunnel: [w681] -> w663 mode=indexing
        tunnel: w662 -> [w680]
        tunnel: w660 -> [w679]
        tunnel: w659 -> [w678]
        tunnel: w657 -> [w677]
        tunnel: w656 -> [w676]
        n250 = for {
          tunnel: w692 -> [w704] mode=indexing
          tunnel: w691 -> [w713]
          tunnel: w690 -> [w716] mode=indexing
          tunnel: w689 -> [w705]
          shift-right: [w723] -> w685
          shift-left: w686 -> [w722]
          shift-right: [w715] -> w687
          shift-left: w688 -> [w717]
          tunnel: w684 -> [w714]
          tunnel: w683 -> [w712]
          tunnel: [w699] -> w682 mode=indexing
          tunnel: [w698] -> w681 mode=indexing
          tunnel: w680 -> [w711]
          tunnel: w679 -> [w695]
          tunnel: w678 -> [w696]
          tunnel: w677 -> [w706]
          tunnel: w676 -> [w703]
          i -> [w697]
          w702 = 2
          w708 = "   "
          n251 = Bundle(w705, w704) -> (w724:cluster{dbl[], dbl[]})  [unwired: 1 in]
          n252 = Number To Fractional String(number=w713, precision (6)=3) -> (F-format string=w719:string)  [unwired: 2 in]
          n253 = Number To Fractional String(number=w716, precision (6)=2) -> (F-format string=w709:string)  [unwired: 2 in]
          n254 = Build Array (concatenate)(w722, w724) -> (w723:cluster{dbl[], dbl[]}[])
          n255 = Index Array(array=w696, index=w697) -> (element=w693:dbl)
          n256 = Index Array(array=w695, index (row)=w697) -> (element=w694:dbl[])  [unwired: 1 in]
          n257 = case shown="2.." w711 {
            tunnel: w694 -> [_ w738 _]
            tunnel: [w735 w738 w739] -> w710
            tunnel: w693 -> [w736 _ _]
            tunnel: w705 -> [w734 _ w740]
            frame ..0 {
              n258 = for {
                tunnel: w736 -> [w737]
                tunnel: [w737] -> w735 mode=indexing
                tunnel: w734 -> [_] mode=indexing
              }
            }
            frame 1 {
            }
            frame 2.. {
              n259 = for {
                tunnel: w740 -> [_] mode=indexing
                tunnel: ["mass constant"] -> w739 mode=indexing
              }
            }
          }
          n260 = call "Dingle fitter.vi"("1/B"=w705, "experiment"=w712, "amp."=w704, "dB/dt"=w714, "T"=w713, "m*"=w710) -> ("gamma"=w699:dbl, "ln [A]"=w698:dbl)  [unwired: 1 out]
          n261 = Number To Fractional String(number=w699, precision (6)=w702) -> (F-format string=w701:string)  [unwired: 2 in]
          n262 = Number To Fractional String(number=w698, precision (6)=w702) -> (F-format string=w700:string)  [unwired: 2 in]
          n263 = Concatenate Strings(w719, w708, w709, w708, w701, w708, w700) -> (w707:string)
          n264 = case shown="True" w703 {
            tunnel: w706 -> [_ w730]
            tunnel: w707 -> [_ w728]
            tunnel: w705 -> [_ w727]
            tunnel: w714 -> [_ w726]
            tunnel: w704 -> [_ w725]
            frame False {
            }
            frame True {
              n265 = Concatenate Strings("Save amp.& dB/dt vs.1/B for T...ln[A]  ", w728) -> (w729:string)
              n266 = Build Array(w727, w726, w725) -> (w732:dbl[][])
              n267 = Transpose 2D Array(2D array=w732) -> (transposed array=w731:dbl[][])
              n268 = call "Write To Spreadsheet File2.vi"("dialogue"=w729, "format (%.3f)"=w730, "2D data"=w731) -> ()  [unwired: 5 in, 1 out]
            }
          }
          n269 = Concatenate Strings(w717, "\r", w707) -> (w715:string)
        }
      }
      "fitted gamma" <- w664
      "fitted intercept" <- w663
      n270 = case shown="True" w654 {
        tunnel: w655 -> [_ w674]
        tunnel: TRUE -> [_ w673]
        frame False {
        }
        frame True {
          n271 = call "Write Characters To File2.vi"("convert eol? (no:F)"=w673, "prompt"="Save parameters?", "character string"=w674) -> ()  [unwired: 2 in, 1 out]
        }
      }
    }
  }
  "plotted data" <- w19
  "plot parameters" <- w15
